vi "cal_main_node_pos.vi"(0 "Last Function Ref":refnum<vi>, 5 "Last Function Position":cluster{"Left":i32, "Top":i32}, 9 "Offset":i32, 11 "error in (no error)":errorcluster) -> (4 "Last Function Ref Out":refnum<vi>, 6 "BD Position":cluster{"Left":i32, "Top":i32}, 15 "error out":errorcluster)   [LabVIEW 2018]
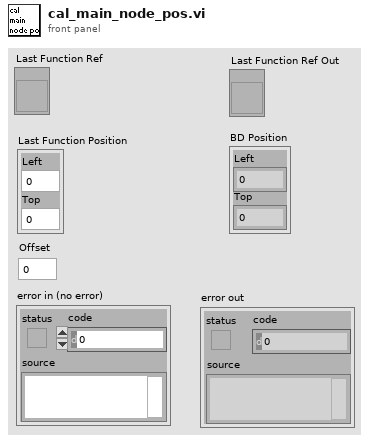
[diagram p1: front panel]
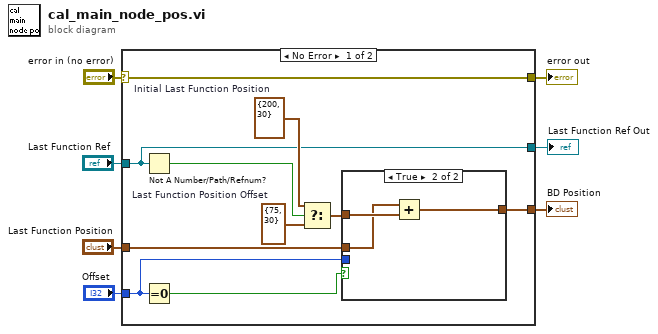
[diagram p0: block diagram]
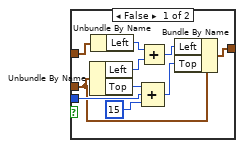
[diagram p2: hidden frame]
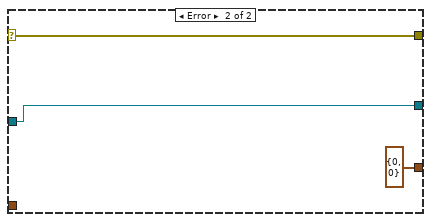
[diagram p3: hidden frame]
diagram:
  n1 = case shown="No Error" "error in (no error)" {
    selector: "error in (no error)" -> [w12 w33]
    tunnel: [w11 cluster{"Left":i32, "Top":i32} {"Left"=0, "Top"=0}] -> w7
    tunnel: "Last Function Position" -> [w16 _]
    tunnel: "Last Function Ref" -> [w8 w31]
    tunnel: [w12 w33] -> w3
    tunnel: "Offset" -> [w9 _]
    tunnel: [w8 w31] -> w1
    frame No Error {
      w13 = cluster{"Left":i32, "Top":i32} {"Left"=200, "Top"=30}  # Initial Last Function Position
      w14 = cluster{"Left":i32, "Top":i32} {"Left"=75, "Top"=30}  # Last Function Position Offset
      n2 = Not A Number/Path/Refnum?(number/path/refnum=w8) -> (NaN/Path/Refnum?=w15:bool)
      n3 = Equal To 0?(x=w9) -> (x = 0?=w10:bool)
      n4 = Select(t=w13, s=w15, f=w14) -> (s? t:f=w17:cluster{"Left":i32, "Top":i32})
      n5 = case shown="True" w10 {
        tunnel: w17 -> [w24 w30]
        tunnel: w16 -> [w22 w29]
        tunnel: [w27 w28] -> w11
        tunnel: w9 -> [w25 _]
        frame False {
          n6 = Unbundle By Name(w22) -> ("Left"=w21:i32, "Top"=w26:i32)
          n7 = Unbundle By Name(w24) -> ("Left"=w20:i32)
          n8 = Add(x=w20, y=w21) -> (x+y=w19:i32)
          n9 = Compound Arithmetic op=ADD(w26, w25, 15 ("value")) -> (w23:i32)
          n10 = Bundle By Name(cluster=w22, "Left"=w19, "Top"=w23) -> (w27:cluster{"Left":i32, "Top":i32})
        }
        frame True {
          n11 = Add(x=w29, y=w30) -> (x+y=w28:cluster{"Left":i32, "Top":i32})
        }
      }
    }
    frame Error {
    }
  }
  "BD Position" <- w7
  "error out" <- w3
  "Last Function Ref Out" <- w1
